vi "Transfer Group Configuration.Get Direction.vi"(11 "Transfer Group Configuration in":refnum<class "Transfer Group Configuration.lvclass">) -> (2 "direction":T1, 3 "Transfer Group Configuration out":refnum<class "Transfer Group Configuration.lvclass">)   [LabVIEW 2017, in "DSF Core.lvlib" / "Transfer Group Configuration.lvclass"]
uses:
  Transfer Group Configuration.lvclass
  DSF Configuration API/Public/Controls/DSF Direction.ctl
  Transfer Group Configuration.lvclass/Transfer Group Configuration.ctl
  DSF Core.lvlib
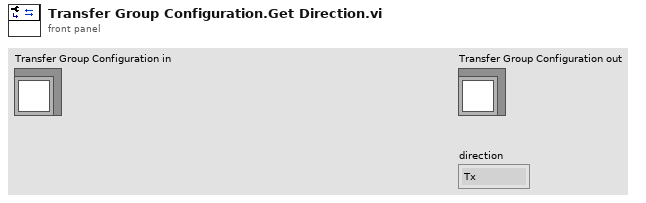
[diagram p1: front panel]
types:
  T1 = typedef "DSF Core.lvlib/DSF Direction.ctl" = enum8{"Tx", "Rx"}
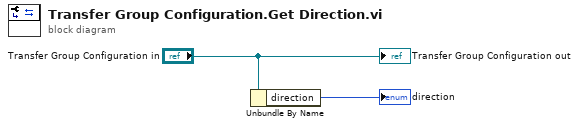
[diagram p0: block diagram]
diagram:
  n1 = Unbundle By Name("Transfer Group Configuration in") -> ("direction"=→"direction":T1)
  "Transfer Group Configuration out" <- "Transfer Group Configuration in"
